vi "Main Page.vi"(8 "error in (no error)":errorcluster, 11 "Node Ptr":T1 format="%.0x") -> (0 "error out":errorcluster)   [LabVIEW 2023, in "Waveform Analog Output System Explorer.lvlib"]
uses:
  Waveform Analog Output System Explorer.lvlib
  <vilib>/NI VeriStand/Custom Device API/Custom Device Item Ref.ctl
  Shared/Constants.vi
  <vilib>/NI VeriStand/Custom Device API/Get Item Property (Double).vi
  <vilib>/NI VeriStand/Custom Device API/Set Item Property (Double).vi
  <vilib>/NI VeriStand/Custom Device API/Get Item Property (String).vi
  <vilib>/NI VeriStand/Custom Device API/Get Item Property (Variant).vi
  <vilib>/NI VeriStand/Custom Device API/Set Item Property (String).vi
  <vilib>/NI VeriStand/Custom Device API/Set Item Property (Variant).vi
  <vilib>/NI VeriStand/Custom Device API/Custom Device API.lvlib
  Shared/Waveform Analog Output Shared.lvlib
panel:
  in  "# of Output Buffers":dbl=2.0
  in  "Start Delay (s)":dbl
  in  "# Samples":dbl=10.0
  in  "Sample Rate (Hz)":dbl=10000.0
  in  "Min Voltage (V)":dbl=-10.0
  in  "Max Voltage (V)":dbl=10.0
  in  "DAQ Name":string caption="DAQ Device Name (Ex: PXI1Slot2)"
  in  "Configure Physical Channels":bool
  in  "Header":cluster{"Section Name":string}={"Section Name"="Waveform Analog Output Configuration"}
  in  "Description":string
  in  "Name":string
  # "Device Settings"
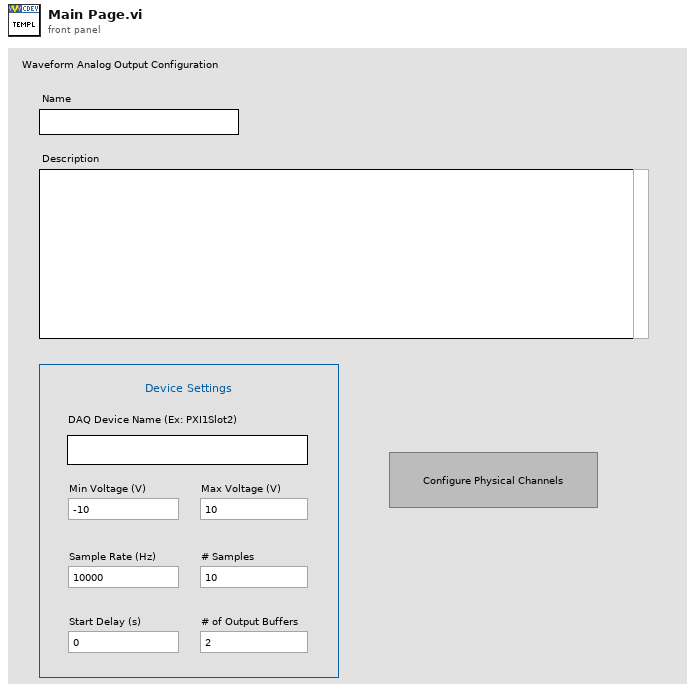
[diagram p1: front panel]
types:
  T1 = typedef "Custom Device API.lvlib/Custom Device Item Ref.ctl" = u64
  T2 = typedef "Custom Device API.lvlib/Custom Device Item Info.ctl" = cluster{"Name":string, "Is Channel":bool, "GUID":string, "Is Waveform":bool}
  T3 = typedef "Custom Device API.lvlib/Custom Device Commands.ctl" = enum16{"Default", "Item renamed", "Shutdown", "Dynamic button pressed"}
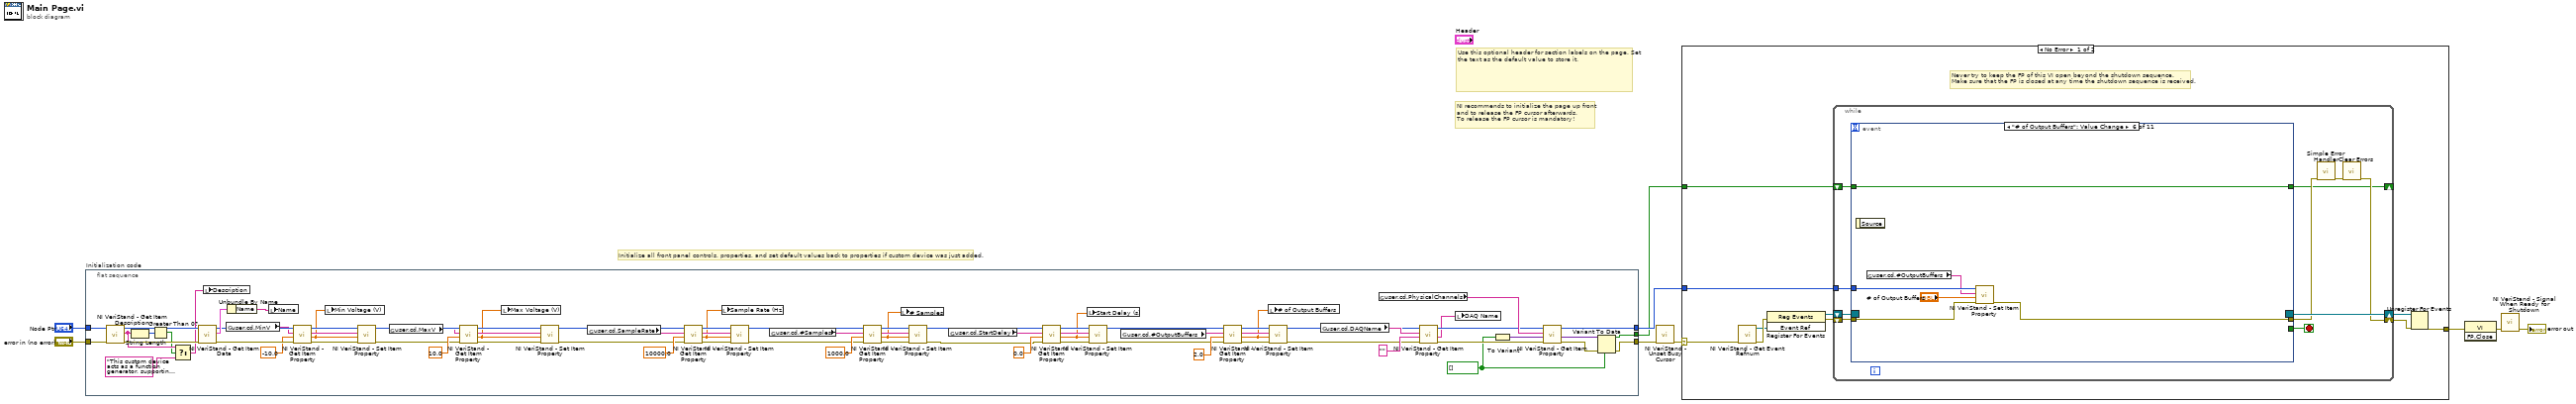
[diagram p0: block diagram]
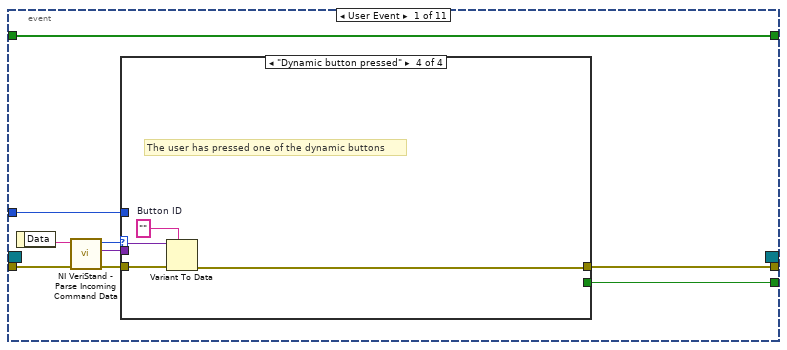
[diagram p2: hidden frame]
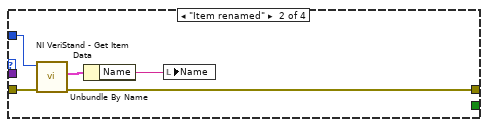
[diagram p4: hidden frame]
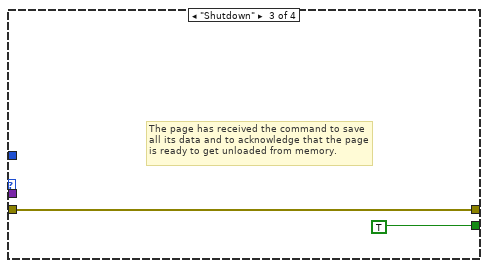
[diagram p5: hidden frame]
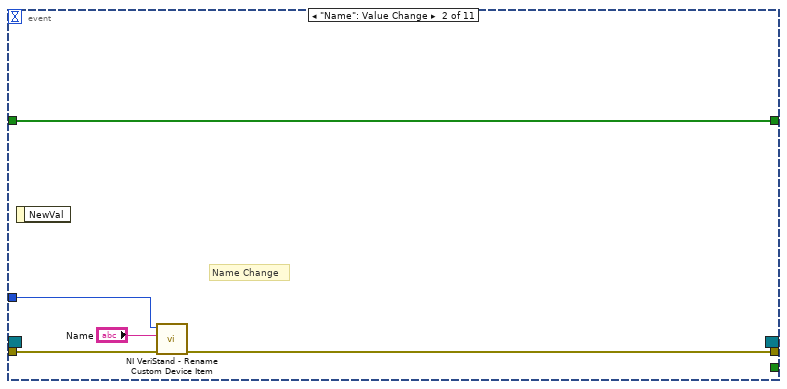
[diagram p6: hidden frame]
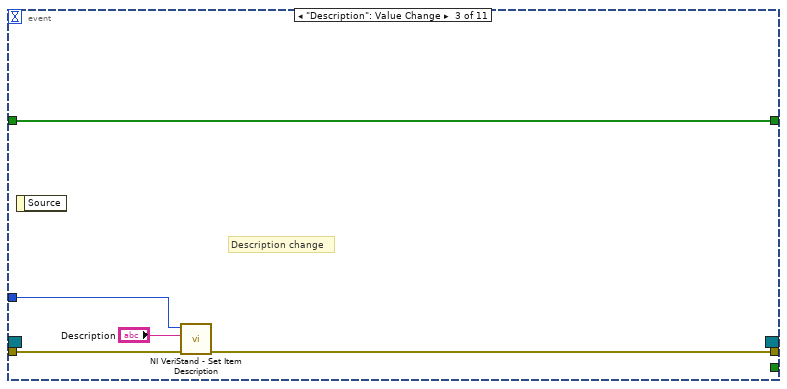
[diagram p7: hidden frame]
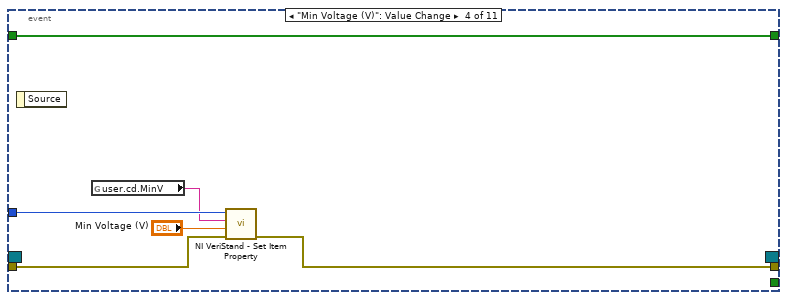
[diagram p8: hidden frame]
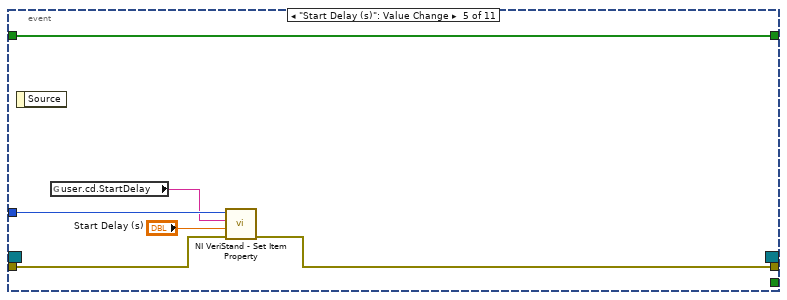
[diagram p9: hidden frame]
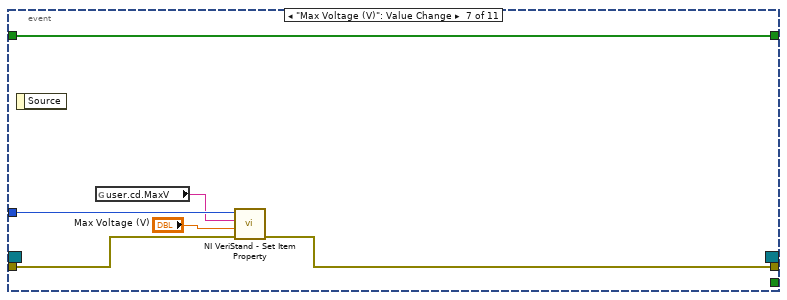
[diagram p10: hidden frame]
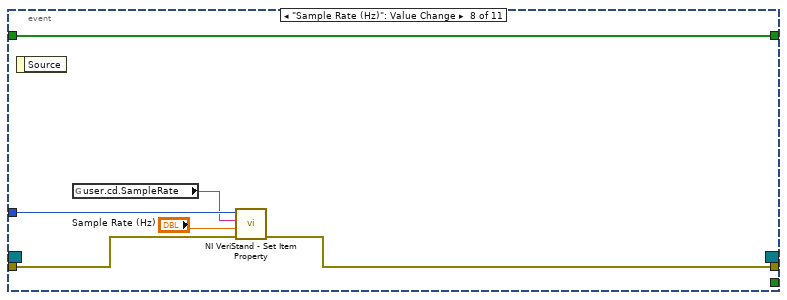
[diagram p11: hidden frame]
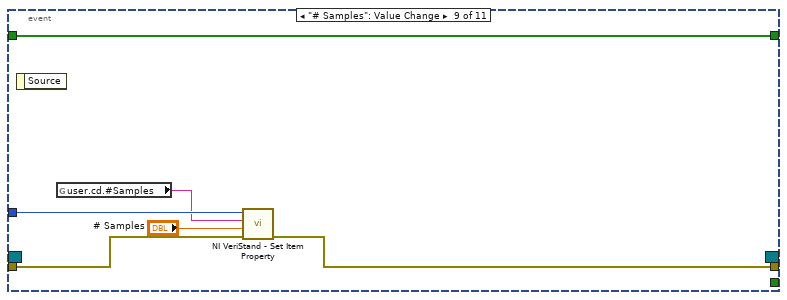
[diagram p12: hidden frame]
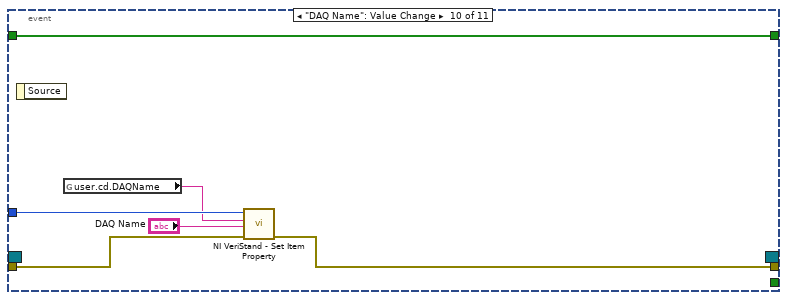
[diagram p13: hidden frame]
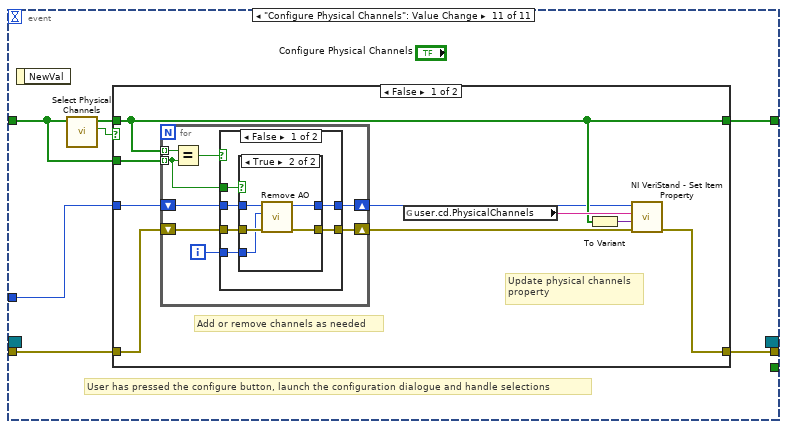
[diagram p14: hidden frame]
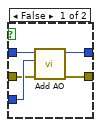
[diagram p15: hidden frame]
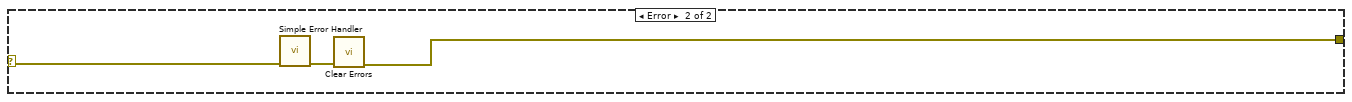
[diagram p18: hidden frame]
diagram:
  # "Initialize all front panel controls, properties, and set default values back to properties if custom device was just added."
  # "Use this optional header for section labels on the page. Set the text as the default value to store it."
  # "NI recommends to initialize the page up front\nand to release the FP cursor afterwards.\nTo release the FP cursor is mandatory!"
  n1 = flat-sequence "Initialization code" {
    tunnel: "error in (no error)" -> [w76]
    tunnel: "Node Ptr" -> [w75]
    tunnel: [w61] -> w5
    tunnel: [w64] -> w2
    tunnel: [w60] -> w1
    frame #0 {
      w54 = bool[] []
      n2 = call <vilib>:"NI VeriStand - Get Item Description.vi"("error in (no error)"=w76, "Item Ref in"=w75) -> ("error out"=w74:errorcluster, "Description"=w28:string, "Item Ref out"=w77:T1)  [unwired: 7 out]
      n3 = String Length(string=w28) -> (length=w29:i32)
      n4 = Greater Than 0?(x=w29) -> (x > 0?=w27:bool)
      n5 = Select(t=w28, s=w27, f="This custom device acts as a function generator, supporting the generation of sine, square, triangle, and sawtooth waveforms. To use this custom device, complete the following:\n1. Enter configuration data below for DAQ name, voltage range, and sampling info.\n2. Press the \"Configure Physical Channels\" button to add or remove AO channels.\n3. Expand the AO# sections to see the tuning channels that are available.  " ("Description")) -> (s? t:f=w30:string)
      n6 = call <vilib>:"NI VeriStand - Get Item Data.vi"("error in (no error)"=w74, "Item Ref in"=w77) -> ("error out"=w70:errorcluster, "Item Info"=w73:T2, "Item Ref out"=w71:T1)  [unwired: 7 out]
      n7 = local write "Description"(w30) -> ()
      n8 = global read "Constants.vi" "user.cd.MinV"() -> (w50:string)
      n9 = Unbundle By Name(w73) -> ("Name"=w72:string)
      n10 = local write "Name"(w72) -> ()
      n11 = call-poly <vilib>:"NI VeriStand - Get Item Property.vi"("error in (no error)"=w70, "Default Value"=-10.0, "Property Name"=w50, "Item Ref in"=w71) -> ("error out"=w48:errorcluster, "Value"=w49:dbl, "Item Ref out"=w51:T1)  [unwired: 4 in, 1 out]
      n12 = local write "Min Voltage (V)"(w49) -> ()
      n13 = call-poly <vilib>:"NI VeriStand - Set Item Property.vi"("error in (no error)"=w48, "Value"=w49, "Property Name"=w50, "Item Ref in"=w51) -> ("error out"=w47:errorcluster, "Item Ref out"=w46:T1)  [unwired: 5 in, 1 out]
      n14 = global read "Constants.vi" "user.cd.MaxV"() -> (w42:string)
      n15 = call-poly <vilib>:"NI VeriStand - Get Item Property.vi"("error in (no error)"=w47, "Default Value"=10.0, "Property Name"=w42, "Item Ref in"=w46) -> ("error out"=w66:errorcluster, "Value"=w41:dbl, "Item Ref out"=w44:T1)  [unwired: 4 in, 1 out]
      n16 = local write "Max Voltage (V)"(w41) -> ()
      n17 = call-poly <vilib>:"NI VeriStand - Set Item Property.vi"("error in (no error)"=w66, "Value"=w41, "Property Name"=w42, "Item Ref in"=w44) -> ("error out"=w45:errorcluster, "Item Ref out"=w43:T1)  [unwired: 5 in, 1 out]
      n18 = global read "Constants.vi" "user.cd.SampleRate"() -> (w39:string)
      n19 = call-poly <vilib>:"NI VeriStand - Get Item Property.vi"("error in (no error)"=w45, "Default Value"=10000.0, "Property Name"=w39, "Item Ref in"=w43) -> ("error out"=w65:errorcluster, "Value"=w38:dbl, "Item Ref out"=w40:T1)  [unwired: 4 in, 1 out]
      n20 = local write "Sample Rate (Hz)"(w38) -> ()
      n21 = call-poly <vilib>:"NI VeriStand - Set Item Property.vi"("error in (no error)"=w65, "Value"=w38, "Property Name"=w39, "Item Ref in"=w40) -> ("error out"=w33:errorcluster, "Item Ref out"=w34:T1)  [unwired: 5 in, 1 out]
      n22 = global read "Constants.vi" "user.cd.#Samples"() -> (w32:string)
      n23 = call-poly <vilib>:"NI VeriStand - Get Item Property.vi"("error in (no error)"=w33, "Default Value"=1000.0, "Property Name"=w32, "Item Ref in"=w34) -> ("error out"=w36:errorcluster, "Value"=w31:dbl, "Item Ref out"=w37:T1)  [unwired: 4 in, 1 out]
      n24 = local write "# Samples"(w31) -> ()
      n25 = call-poly <vilib>:"NI VeriStand - Set Item Property.vi"("error in (no error)"=w36, "Value"=w31, "Property Name"=w32, "Item Ref in"=w37) -> ("error out"=w20:errorcluster, "Item Ref out"=w21:T1)  [unwired: 5 in, 1 out]
      n26 = global read "Constants.vi" "user.cd.StartDelay"() -> (w25:string)
      n27 = call-poly <vilib>:"NI VeriStand - Get Item Property.vi"("error in (no error)"=w20, "Default Value"=0.0, "Property Name"=w25, "Item Ref in"=w21) -> ("error out"=w23:errorcluster, "Value"=w19:dbl, "Item Ref out"=w22:T1)  [unwired: 4 in, 1 out]
      n28 = local write "Start Delay (s)"(w19) -> ()
      n29 = call-poly <vilib>:"NI VeriStand - Set Item Property.vi"("error in (no error)"=w23, "Value"=w19, "Property Name"=w25, "Item Ref in"=w22) -> ("error out"=w13:errorcluster, "Item Ref out"=w14:T1)  [unwired: 5 in, 1 out]
      n30 = global read "Constants.vi" "user.cd.#OutputBuffers"() -> (w15:string)
      n31 = call-poly <vilib>:"NI VeriStand - Get Item Property.vi"("error in (no error)"=w13, "Default Value"=2.0, "Property Name"=w15, "Item Ref in"=w14) -> ("error out"=w17:errorcluster, "Value"=w12:dbl, "Item Ref out"=w18:T1)  [unwired: 4 in, 1 out]
      n32 = local write "# of Output Buffers"(w12) -> ()
      n33 = call-poly <vilib>:"NI VeriStand - Set Item Property.vi"("error in (no error)"=w17, "Value"=w12, "Property Name"=w15, "Item Ref in"=w18) -> ("error out"=w10:errorcluster, "Item Ref out"=w11:T1)  [unwired: 5 in, 1 out]
      n34 = global read "Constants.vi" "user.cd.DAQName"() -> (w58:string)
      n35 = global read "Constants.vi" "user.cd.PhysicalChannels"() -> (w63:string)
      n36 = call-poly <vilib>:"NI VeriStand - Get Item Property.vi"("error in (no error)"=w10, "Default Value"="", "Property Name"=w58, "Item Ref in"=w11) -> ("error out"=w56:errorcluster, "Value"=w55:string, "Item Ref out"=w59:T1)  [unwired: 4 in, 1 out]
      n37 = local write "DAQ Name"(w55) -> ()
      n38 = To Variant(anything=w54) -> (Variant=w62:variant)
      n39 = call-poly <vilib>:"NI VeriStand - Get Item Property.vi"("error in (no error)"=w56, "Default Value"=w62, "Property Name"=w63, "Item Ref in"=w59) -> ("error out"=w53:errorcluster, "Value"=w52:variant, "Item Ref out"=w64:T1)  [unwired: 4 in, 1 out]
      n40 = Variant To Data(error in=w53, type=w54, Variant=w52) -> (data=w60:bool[], error out=w61:errorcluster)
    }
  }
  n41 = call <vilib>:"NI VeriStand - Unset Busy Cursor.vi"("error in (no error)"=w5) -> ("error out"=w4:errorcluster)  [unwired: 10 out]
  n42 = case shown="No Error" w4 {
    selector: w4 -> [w79 w217]
    tunnel: [w84 w215] -> w9
    tunnel: w2 -> [w80 _]
    tunnel: w1 -> [w78 _]
    frame No Error {
      # "Never try to keep the FP of this VI open beyond the shutdown sequence.\nMake sure that the FP is closed at any time the shutdown sequence is received."
      n43 = call <vilib>:"NI VeriStand - Get Event Refnum.vi"("error in (no error)"=w79) -> ("error out"=w87:errorcluster, "Event Ref"=w83:refnum<user-event>)  [unwired: 9 out]
      n44 = register-events(error in=w87, w83) -> (reference out=w81:refnum<event-registration>, error out=w82:errorcluster)  [unwired: 1 in]
      n45 = while {
        tunnel: w80 -> [w93]
        shift-right: [w90] -> w85
        shift-left: w82 -> [w96]
        shift-right: [w97] -> w86
        shift-left: w81 -> [w95]
        shift-right: [w88] -> _
        shift-left: w78 -> [w89]
        stop <- w94 stop-if-true
        n46 = event shown="[5] \"# of Output Buffers\": Value Change" {
          selector: w95 -> [_ _ _ _ _ _ _ _ _ _ _]
          dyn-events: [_ _ _ _ _ _ _ _ _ _ _] -> w97
          timeout: _ -> [_ _ _ _ _ _ _ _ _ _ _]
          tunnel: w96 -> [w106 w123 w127 w133 w139 w145 w151 w157 w163 w169 w177]
          tunnel: [w102 _ _ _ _ _ _ _ _ _ _] -> w94
          tunnel: [w101 w122 w126 w130 w137 w143 w149 w155 w161 w167 w176] -> w92
          tunnel: w93 -> [w100 w121 w128 w134 w140 w146 w152 w158 w164 w170 w175]
          tunnel: w89 -> [w98 w119 w124 w129 w136 w142 w147 w153 w160 w166 w171]
          tunnel: [w98 w119 w124 w129 w136 w142 w147 w153 w160 w166 w173] -> w88
          event User Event {
            n47 = event-data() -> ("Data"=w105:string)  [unwired: 1 out]
            n48 = call <vilib>:"NI VeriStand - Parse Incoming Command Data.vi"("error in (no error)"=w106, "Incoming data"=w105) -> ("error out"=w104:errorcluster, "Outgoing data"=w99:variant, "Action"=w103:T3)  [unwired: 7 out]
            n49 = case shown="\"Dynamic button pressed\"" w103 {
              tunnel: w104 -> [w107 w112 w113 w118]
              tunnel: [_ _ TRUE _] -> w102
              tunnel: [w107 w109 w113 w115] -> w101
              tunnel: w100 -> [_ w111 _ _]
              tunnel: w99 -> [_ _ _ w117]
              frame "Default", Default {
              }
              frame "Item renamed" {
                n50 = call <vilib>:"NI VeriStand - Get Item Data.vi"("error in (no error)"=w112, "Item Ref in"=w111) -> ("error out"=w109:errorcluster, "Item Info"=w110:T2)  [unwired: 8 out]
                n51 = Unbundle By Name(w110) -> ("Name"=w108:string)
                n52 = local write "Name"(w108) -> ()
              }
              frame "Shutdown" {
                # "The page has received the command to save all its data and to acknowledge that the page is ready to get unloaded from memory."
              }
              frame "Dynamic button pressed" {
                w116 = ""  # Button ID
                # "The user has pressed one of the dynamic buttons"
                n53 = Variant To Data(error in=w118, type=w116, Variant=w117) -> (error out=w115:errorcluster)  [unwired: 1 out]
              }
            }
          }
          event "Name": Value Change {
            # "Name Change"
            n54 = event-data() -> ()  [unwired: 2 out]
            n55 = call <vilib>:"NI VeriStand - Rename Custom Device Item.vi"("error in (no error)"=w123, "New Name"="Name", "Item Ref in"=w121) -> ("error out"=w122:errorcluster)  [unwired: 1 in, 7 out]
          }
          event "Description": Value Change {
            # "Description change"
            n56 = event-data() -> ()  [unwired: 2 out]
            n57 = call <vilib>:"NI VeriStand - Set Item Description.vi"("error in (no error)"=w127, "Description"="Description", "Item Ref in"=w128) -> ("error out"=w126:errorcluster)  [unwired: 8 out]
          }
          event "Min Voltage (V)": Value Change {
            n58 = event-data() -> ()  [unwired: 2 out]
            n59 = global read "Constants.vi" "user.cd.MinV"() -> (w132:string)
            n60 = call-poly <vilib>:"NI VeriStand - Set Item Property.vi"("error in (no error)"=w133, "Value"="Min Voltage (V)", "Property Name"=w132, "Item Ref in"=w134) -> ("error out"=w130:errorcluster)  [unwired: 5 in, 2 out]
          }
          event "Start Delay (s)": Value Change {
            n61 = event-data() -> ()  [unwired: 2 out]
            n62 = global read "Constants.vi" "user.cd.StartDelay"() -> (w138:string)
            n63 = call-poly <vilib>:"NI VeriStand - Set Item Property.vi"("error in (no error)"=w139, "Value"="Start Delay (s)", "Property Name"=w138, "Item Ref in"=w140) -> ("error out"=w137:errorcluster)  [unwired: 5 in, 2 out]
          }
          event "# of Output Buffers": Value Change {
            n64 = event-data() -> ()  [unwired: 2 out]
            n65 = global read "Constants.vi" "user.cd.#OutputBuffers"() -> (w144:string)
            n66 = call-poly <vilib>:"NI VeriStand - Set Item Property.vi"("error in (no error)"=w145, "Value"="# of Output Buffers", "Property Name"=w144, "Item Ref in"=w146) -> ("error out"=w143:errorcluster)  [unwired: 5 in, 2 out]
          }
          event "Max Voltage (V)": Value Change {
            n67 = event-data() -> ()  [unwired: 2 out]
            n68 = global read "Constants.vi" "user.cd.MaxV"() -> (w150:string)
            n69 = call-poly <vilib>:"NI VeriStand - Set Item Property.vi"("error in (no error)"=w151, "Value"="Max Voltage (V)", "Property Name"=w150, "Item Ref in"=w152) -> ("error out"=w149:errorcluster)  [unwired: 5 in, 2 out]
          }
          event "Sample Rate (Hz)": Value Change {
            n70 = event-data() -> ()  [unwired: 2 out]
            n71 = global read "Constants.vi" "user.cd.SampleRate"() -> (w156:string)
            n72 = call-poly <vilib>:"NI VeriStand - Set Item Property.vi"("error in (no error)"=w157, "Value"="Sample Rate (Hz)", "Property Name"=w156, "Item Ref in"=w158) -> ("error out"=w155:errorcluster)  [unwired: 5 in, 2 out]
          }
          event "# Samples": Value Change {
            n73 = event-data() -> ()  [unwired: 2 out]
            n74 = global read "Constants.vi" "user.cd.#Samples"() -> (w162:string)
            n75 = call-poly <vilib>:"NI VeriStand - Set Item Property.vi"("error in (no error)"=w163, "Value"="# Samples", "Property Name"=w162, "Item Ref in"=w164) -> ("error out"=w161:errorcluster)  [unwired: 5 in, 2 out]
          }
          event "DAQ Name": Value Change {
            n76 = event-data() -> ()  [unwired: 2 out]
            n77 = global read "Constants.vi" "user.cd.DAQName"() -> (w168:string)
            n78 = call-poly <vilib>:"NI VeriStand - Set Item Property.vi"("error in (no error)"=w169, "Value"="DAQ Name", "Property Name"=w168, "Item Ref in"=w170) -> ("error out"=w167:errorcluster)  [unwired: 5 in, 2 out]
          }
          event "Configure Physical Channels": Value Change {
            # "User has pressed the configure button, launch the configuration dialogue and handle selections"
            n79 = event-data() -> ()  [unwired: 2 out]
            n80 = call "Select Physical Channels.vi"("Physical Channels In"=w171) -> ("Cancelled?"=w172:bool, "Physical Channels Out"=w174:bool[])  [unwired: 9 in]
            n81 = case shown="False" w172 {
              tunnel: w177 -> [w179 w213]
              tunnel: [w186 w213] -> w176
              tunnel: w175 -> [w181 _]
              tunnel: w174 -> [w183 w214]
              tunnel: [w183 w214] -> w173
              tunnel: w171 -> [w182 _]
              frame False {
                # "Update physical channels\nproperty"
                # "Add or remove channels as needed"
                n82 = for {
                  tunnel: w183 -> [w194] mode=indexing
                  tunnel: w182 -> [w190] mode=indexing
                  shift-right: [w188] -> w180
                  shift-left: w181 -> [w192]
                  shift-right: [w187] -> w178
                  shift-left: w179 -> [w191]
                  i -> [w189]
                  n83 = Equal?(x=w194, y=w190) -> (x = y?=w193:bool)
                  n84 = case shown="False" w193 {
                    tunnel: w192 -> [w198 w212]
                    tunnel: w191 -> [w197 w211]
                    tunnel: w190 -> [w200 _]
                    tunnel: w189 -> [w199 _]
                    tunnel: [w196 w212] -> w188
                    tunnel: [w195 w211] -> w187
                    frame False {
                      n85 = case shown="True" w200 {
                        tunnel: w199 -> [w204 w209]
                        tunnel: w198 -> [w205 w208]
                        tunnel: w197 -> [w203 w210]
                        tunnel: [w202 w206] -> w196
                        tunnel: [w201 w207] -> w195
                        frame False {
                          n86 = call "Add AO.vi"("error in (no error)"=w203, "Physical Channel Number"=w204, "Device Item Ref in"=w205) -> ("error out"=w201:errorcluster, "Parent Ref out"=w202:T1)  [unwired: 7 in]
                        }
                        frame True {
                          n87 = call "Remove AO.vi"("error in (no error)"=w210, "Iteration"=w209, "Item Ref in"=w208) -> ("error out"=w207:errorcluster, "Item Ref out"=w206:T1)  [unwired: 7 in]
                        }
                      }
                    }
                    frame True {
                    }
                  }
                }
                n88 = global read "Constants.vi" "user.cd.PhysicalChannels"() -> (w185:string)
                n89 = To Variant(anything=w183) -> (Variant=w184:variant)
                n90 = call-poly <vilib>:"NI VeriStand - Set Item Property.vi"("error in (no error)"=w178, "Value"=w184, "Property Name"=w185, "Item Ref in"=w180) -> ("error out"=w186:errorcluster)  [unwired: 5 in, 2 out]
              }
              frame True {
              }
            }
          }
        }
        n91 = call <vilib>:"Simple Error Handler.vi"("error in (no error)"=w92) -> ("error out"=w91:errorcluster)  [unwired: 1 in, 7 out]
        n92 = call <vilib>:"Clear Errors.vi"("error in (no error)"=w91) -> ("error out"=w90:errorcluster)  [unwired: 1 in, 5 out]
      }
      n93 = Unregister For Events(event registration refnum=w86, error in=w85) -> (error out=w84:errorcluster)
    }
    frame Error {
      n94 = call <vilib>:"Simple Error Handler.vi"("error in (no error)"=w217) -> ("error out"=w216:errorcluster)  [unwired: 1 in, 7 out]
      n95 = call <vilib>:"Clear Errors.vi"("error in (no error)"=w216) -> ("error out"=w215:errorcluster)  [unwired: 1 in, 5 out]
    }
  }
  n96 = invoke class="VI" method="FP.Close"(error in=w9) -> (error out=w8:errorcluster)  [unwired: 2 in, 2 out]
  n97 = call <vilib>:"NI VeriStand - Signal When Ready for Shutdown.vi"("error in (no error)"=w8) -> ("error out"=→"error out":errorcluster)  [unwired: 10 out]
